vi "Load DAQmx Insruments.vi"() -> (3 "Instruments":refnum<class "Dynamic Instrument.lvclass">[](array[class]))   [LabVIEW 2016]
uses:
  Dynamic Instrument/Dynamic Instrument/Dynamic Instrument.lvclass
  DAQmx Digitizer/DAQmx Digitizer.lvclass
  C:/github/NHMFL_Core/Libraries/NI-DAQ/Dynamic Load/Dynamic Instrument/Dynamic Instrument/Dynamic Instrument.lvclass
  Dynamic Instrument/Dynamic Instrument/Dynamic Instrument.lvclass/Dynamic Instrument.ctl
  Dynamic Instrument/Dynamic Instrument/Write Instrument Name.vi
  <resource>/objmgr/daqmx.rc
panel:
  out "Device names":tag[](array[tag])
  out "Error Out":errorcluster
  in  "Error In":errorcluster
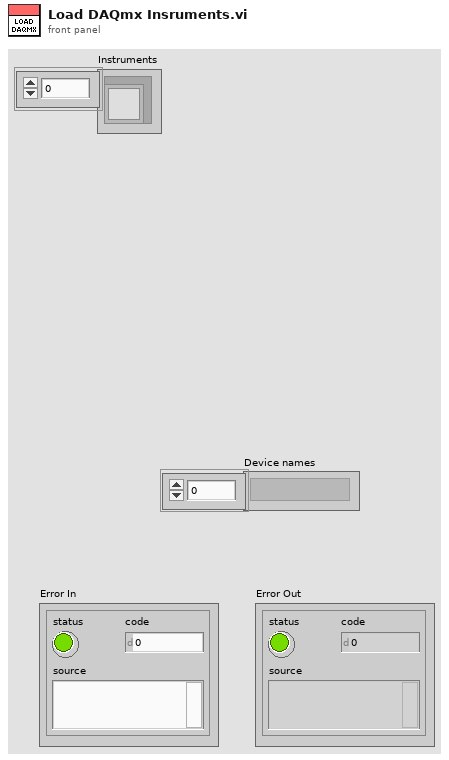
[diagram p1: front panel]
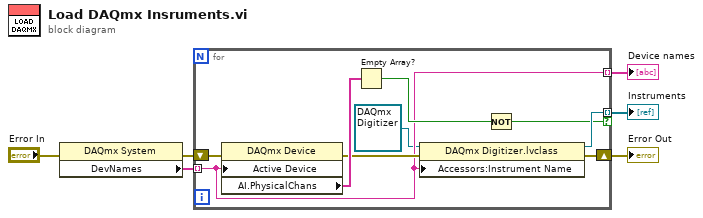
[diagram p0: block diagram]
diagram:
  n1 = property class="DAQmx System"(error in="Error In") -> (error out=w5:errorcluster, "DevNames"=w6:tag[])  [unwired: 1 in, 1 out]
  n2 = for {
    tunnel: w6 -> [w8] mode=indexing
    shift-right: [w12] -> w3
    shift-left: w5 -> [w15]
    tunnel: [w11] -> w1 mode=indexing if=w9
    tunnel: [w8] -> w2 mode=indexing
    n3 = property class="DAQmx Device"(error in=w15, "Active Device"=w8) -> (error out=w13:errorcluster, "AI.PhysicalChans"=w14:tag[])  [unwired: 1 in, 1 out]
    n4 = Empty Array?(array=w14) -> (empty?=w10:bool)
    n5 = property class="DAQmx Digitizer.lvclass"(reference=refnum<class "DAQmx Digitizer.lvclass"> refnum ("DAQmx Digitizer.lvlib:DAQmx Digitizer.lvclass"), error in=w13, "Accessors:Instrument Name"=w8) -> (reference out=w11:refnum<class "DAQmx Digitizer.lvclass">, error out=w12:errorcluster)
    n6 = Not(x=w10) -> (.not. x?=w9:bool)
  }
  "Instruments" <- w1
  "Error Out" <- w3
  "Device names" <- w2
